vi "LabView360-5-FileIO.vi"() -> ()   [LabVIEW 2017]
panel:
  in  "文件路径（使用对话框）":path
  out "电子表格字符串":string
  out "数组":dbl[][](array[numeric])
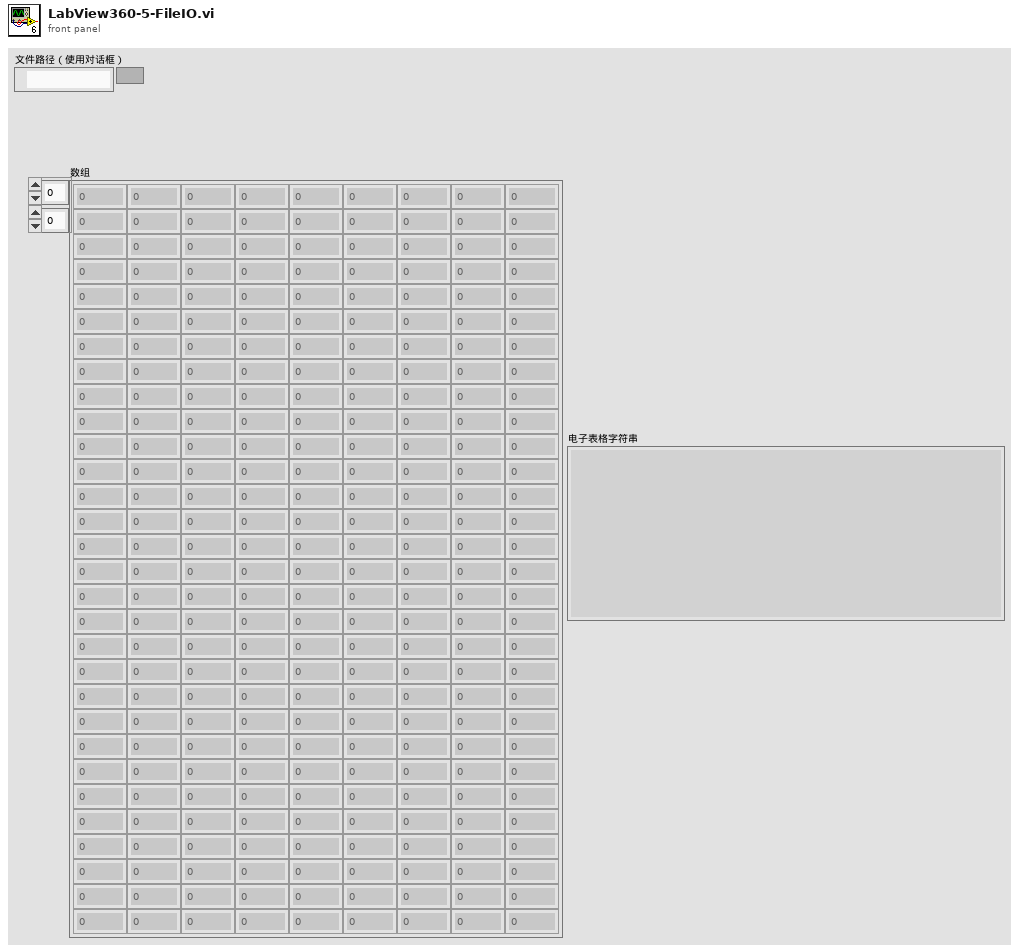
[diagram p1: front panel]
types:
  T1 = enum16{"open", "replace", "create", "open or create", "replace or create", "replace or create with confirmation"}
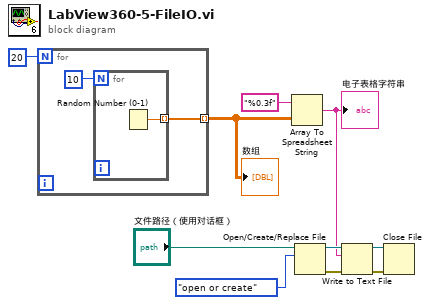
[diagram p0: block diagram]
diagram:
  n1 = for {
    N: 20 -> [_]
    tunnel: [w11] -> w9 mode=indexing
    n2 = for {
      N: 10 -> [_]
      tunnel: [w13] -> w11 mode=indexing
      n3 = Random Number (0-1)() -> (number: 0 to 1=w13:dbl)
    }
  }
  "数组" <- w9
  n4 = Array To Spreadsheet String(array=w9, 3:"%0.3f" ("格式字符串")) -> (spreadsheet string=w1:string)  [unwired: 1 in]
  "电子表格字符串" <- w1
  n5 = Open/Create/Replace File(file path (use dialog)="文件路径（使用对话框）", operation (0:open)=T1."open or create" ("操作(0:open)")) -> (refnum out=w5:refnum<file>, error out=w4:errorcluster)  [unwired: 4 in, 1 out]
  n6 = Write to Text File(file (use dialog)=w5, text=w1, error in=w4) -> (refnum out=w2:refnum<file>, error out=w3:errorcluster)  [unwired: 1 in, 1 out]
  n7 = Close File(refnum=w2, error in=w3) -> ()  [unwired: 2 out]
